vi "Inverse Error Function Complement.vi"(3 "x":dbl) -> (1 "inverfc(x)":dbl)   [LabVIEW 2020, in "NI_AAL_MathFunc.lvlib"]
doc: "Computes the inverse of the complementary error function associated with a normal distribution."
uses:
  <vilib>/gmath/NI_AAL_MathFunc.lvlib
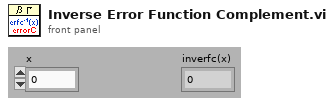
[diagram p1: front panel]
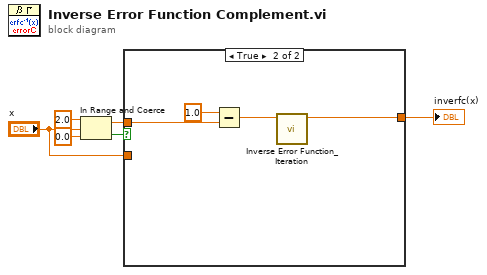
[diagram p0: block diagram]
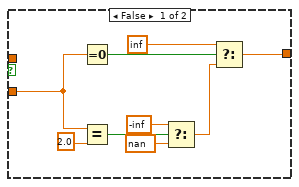
[diagram p2: hidden frame]
diagram:
  n1 = In Range and Coerce(upper limit=2.0, x="x", lower limit=0.0) -> (coerced(x)=w2:dbl, In Range?=w5:bool)
  n2 = case shown="True" w5 {
    tunnel: w2 -> [_ w19]
    tunnel: [w8 w16] -> w6
    tunnel: "x" -> [w7 _]
    frame False {
      n3 = Equal To 0?(x=w7) -> (x = 0?=w11:bool)
      n4 = Equal?(x=w7, y=2.0) -> (x = y?=w14:bool)
      n5 = Select(t=-inf, s=w14, f=nan) -> (s? t:f=w10:dbl)
      n6 = Select(t=inf, s=w11, f=w10) -> (s? t:f=w8:dbl)
    }
    frame True {
      n7 = Subtract(x=1.0, y=w19) -> (x-y=w17:dbl)
      n8 = call <vilib>:"Inverse Error Function_Iteration.vi"("x"=w17) -> ("erfinv(x)"=w16:dbl)  [unwired: 10 in]
    }
  }
  "inverfc(x)" <- w6
